vi "Import QD Shortcuts.vi"() -> ()   [LabVIEW 2017, in "NEVSTOP_QuickDrop.lvlib"]
doc: "Backs up LabVIEW.ini, shows the tokens of a selected .iniToken file in a chooser dialog and writes the chosen tokens into LabVIEW.ini."
uses:
  NEVSTOP_QuickDrop.lvlib
  XTwoColSelector.v1.1.llb/XTwoColumnSelector.xctl
panel:
  in  "XTwoColumnSelector":string[](xcontrol)
  in  "System OK Button":bool
  in  "System Cancel Button":bool
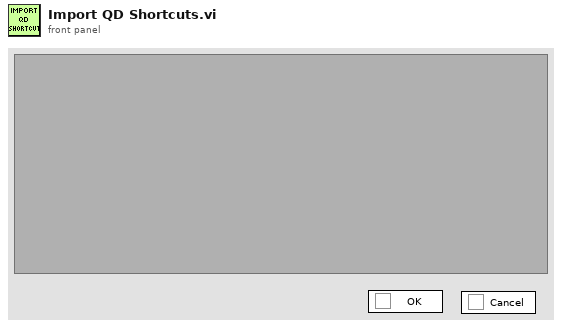
[diagram p1: front panel]
types:
  T1 = typedef "Def-IniTokenCluster.ctl" = cluster{"Session":string, "Token":string, "ListConnector":string}
  T2 = cluster{"IniTokenCluster":T1, "Items":string[]}[]
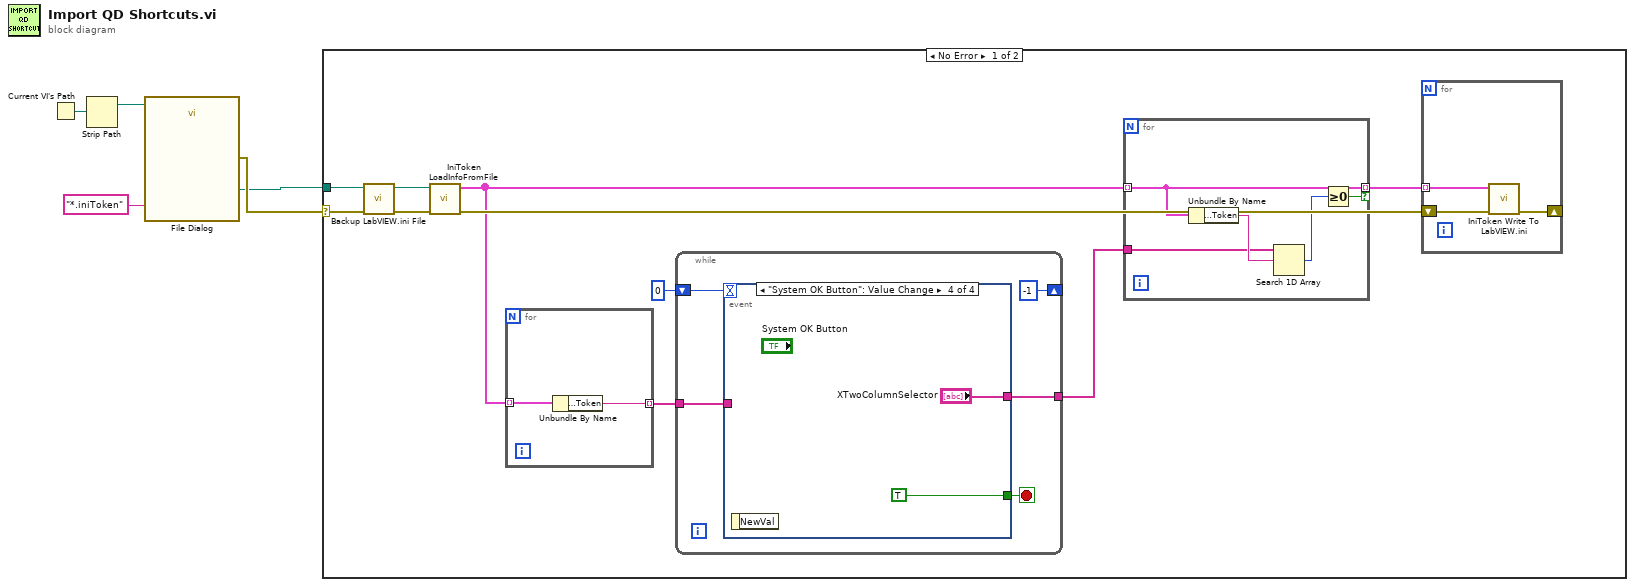
[diagram p0: block diagram]
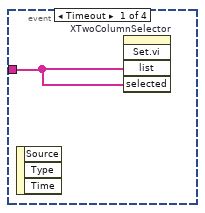
[diagram p2: hidden frame]
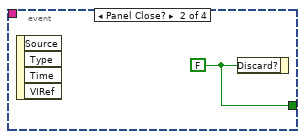
[diagram p3: hidden frame]
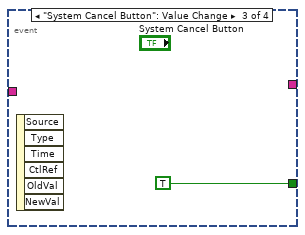
[diagram p4: hidden frame]
diagram:
  n1 = Current VI's Path() -> (path=w2:path)
  n2 = Strip Path(path=w2) -> (stripped path=w1:path)  [unwired: 1 out]
  n3 = call "File Dialog"("start path"=w1, "pattern (all files)"="*.iniToken") -> ("selected path"=w3:path, "error out"=w4:errorcluster)  [unwired: 10 in, 2 out]
  n4 = case shown="No Error" w4 {
    selector: w4 -> [w12 _]
    tunnel: w3 -> [w13 _]
    frame No Error {
      n5 = call "Backup LabVIEW.ini File.vi"("error in (no error)"=w12) -> ("error out"=w6:errorcluster)  [unwired: 9 in, 1 out]
      n6 = call "IniToken LoadInfoFromFile.vi"("error in (no error)"=w6, "Path"=w13) -> ("error out"=w11:errorcluster, "Array"=w9:T2)  [unwired: 8 in]
      n7 = for {
        tunnel: w9 -> [w21] mode=indexing
        tunnel: [w20] -> w10 mode=indexing
        n8 = Unbundle By Name(w21) -> ("IniTokenCluster.Token"=w20:string)
      }
      n9 = while {
        tunnel: [w28] -> w7
        shift-right: [-1] -> _
        shift-left: 0 -> [w27]
        tunnel: w10 -> [w25]
        stop <- w29 stop-if-true
        n10 = event shown="[3] \"System OK Button\": Value Change" {
          selector: _ -> [_ _ _ _]
          dyn-events: _ -> [_ _ _ _]
          timeout: w27 -> [_ _ _ _]
          tunnel: [_ w31 TRUE ("Discard?") TRUE ("Discard?")] -> w29
          tunnel: [_ _ _ "XTwoColumnSelector"] -> w28
          tunnel: w25 -> [w30 _ _ _]
          event Timeout {
            n11 = event-data() -> ()  [unwired: 1 in, 3 out]
            n12 = invoke on="XTwoColumnSelector" class="XTwoColumnSelector (strict)" method="Set.vi"("list"=w30, "selected"=w30) -> ()  [unwired: 3 in, 5 out]
          }
          event Panel Close? {
            w31 = FALSE ("Discard?")
            n13 = event-data() -> ()  [unwired: 1 in, 4 out]
            n14 = event-data("Discard?"=w31) -> ()  [unwired: 1 in, 1 out]
          }
          event "System Cancel Button": Value Change {
            n15 = event-data() -> ()  [unwired: 1 in, 6 out]
          }
          event "System OK Button": Value Change {
            n16 = event-data() -> ()  [unwired: 1 in, 1 out]
          }
        }
      }
      n17 = for {
        tunnel: w9 -> [w19] mode=indexing
        tunnel: [w19] -> w8 mode=indexing if=w15
        tunnel: w7 -> [w17]
        n18 = Unbundle By Name(w19) -> ("IniTokenCluster.Token"=w18:string)
        n19 = Search 1D Array(1D array=w17, element=w18) -> (index of element=w16:i32)  [unwired: 1 in]
        n20 = Greater Or Equal To 0?(x=w16) -> (x >= 0?=w15:bool)
      }
      n21 = for {
        tunnel: w8 -> [w24] mode=indexing
        shift-right: [w22] -> _
        shift-left: w11 -> [w23]
        n22 = call "IniToken Write To LabVIEW.ini.vi"("error in (no error)"=w23, "Cluster"=w24) -> ("error out"=w22:errorcluster)  [unwired: 9 in]
      }
    }
    frame Error {
    }
  }
